vi "Main.vi"() -> ()   [LabVIEW 2020]
doc: "This template is for the Queued Message Handler design pattern.\n\nThe Event Handling Loop generates messages based on user interface actions.\n\nThe Message Handling Loop processes messages generated by the Event Handling Loop, or by other messages. The messages are string values, so new messages can be added easily to the Message Cases case structure in the Message Handling Loop. Each message cluster can also provide an optional value for Message Data, which is a variant that can be converted to whatever message-specific data is required."
uses:
  controls/WashIndicators.ctl
  controls/WashOptions.ctl
  controls/UI Data.ctl
  support/Message Queue/Message Queue.lvlib
  support/User Event - Stop/User Event - Stop.lvlib
panel:
  in  "Wash Options":T1
  out "Car Wash Indicators 2":T2
  in  "Car Position Slider":u16(slide) scale=0.0..4.0
  out "Wash Entry":bool
  out "Elapsed Time":dbl format="%<%H:%M:%S>t"
  in  "Start":bool
  in  "Stop":bool
  # "Pre-Soak\nH-P Wash\nL-P Wax\nSpot Free Rinse"
  # "Underbody Wash\nBug Remover"
  # "Tire Shine\nAir Dry"
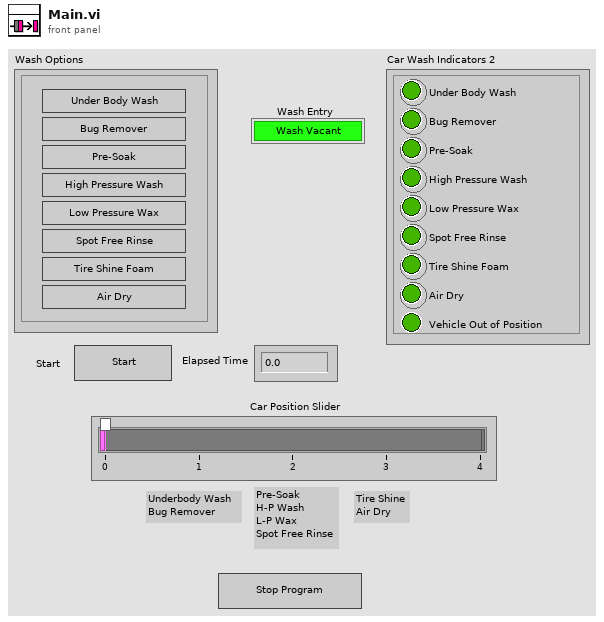
[diagram p1: front panel]
types:
  T1 = typedef "WashOptions.ctl" = cluster{"Bug Remover":bool, "Low Pressure Wax":bool, "High Pressure Wash":bool, "Pre-Soak":bool, "Spot Free Rinse":bool, "Air Dry":bool, "Under Body Wash":bool, "Tire Shine Foam":bool}
  T2 = typedef "WashIndicators.ctl" = cluster{"Bug Remover":bool, "Pre-Soak":bool, "High Pressure Wash":bool, "Spot Free Rinse":bool, "Tire Shine Foam":bool, "Low Pressure Wax":bool, "Vehicle Out of Position":bool, "Air Dry":bool, "Under Body Wash":bool}
  T3 = typedef "UI Data.ctl" = cluster{"Elapsed Time":refnum<vi>, "Wash Entry":refnum<vi>, "Car Position Slider":refnum<vi>, "Wash Options":refnum<vi>, "Car Wash Indicators":refnum<vi>, "Car Wash Indicators 2":T2}
  T4 = typedef "Message Queue.lvlib/All Message Queues.ctl" = cluster{"UI":refnum<queue>, "Status Loop":refnum<queue>}
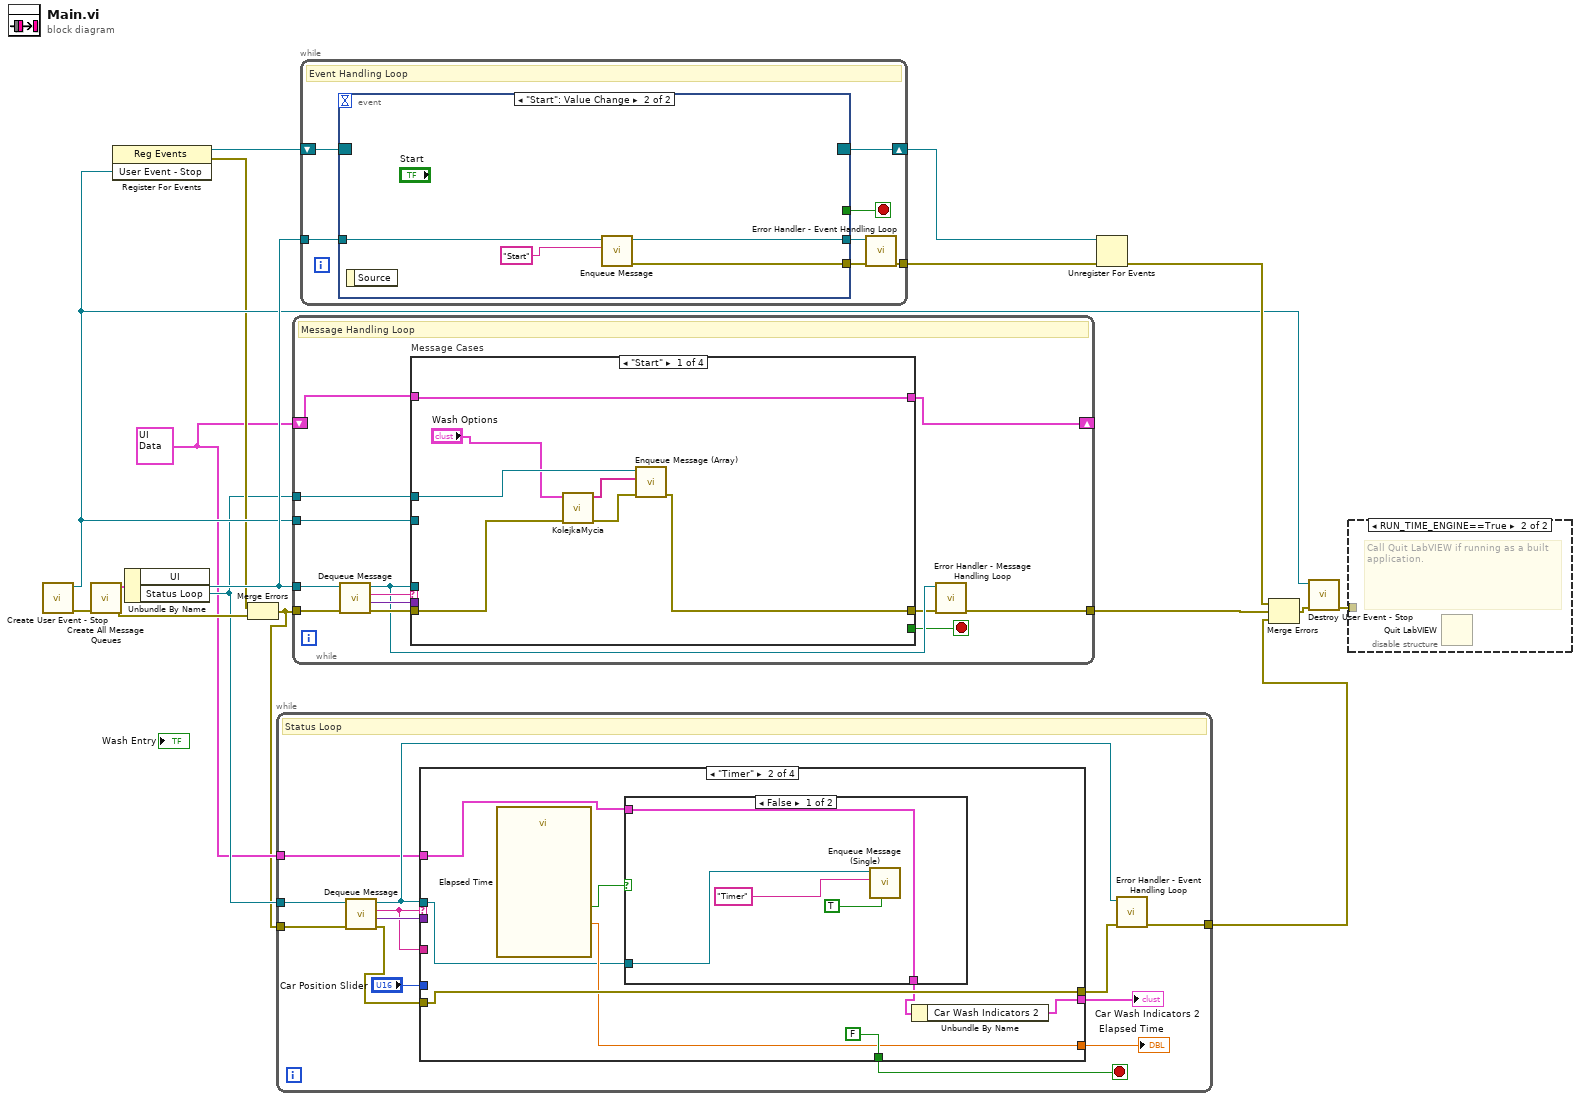
[diagram p0: block diagram]
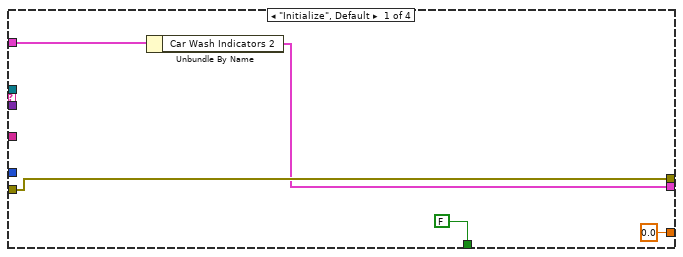
[diagram p2: hidden frame]
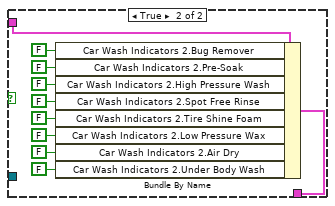
[diagram p3: hidden frame]
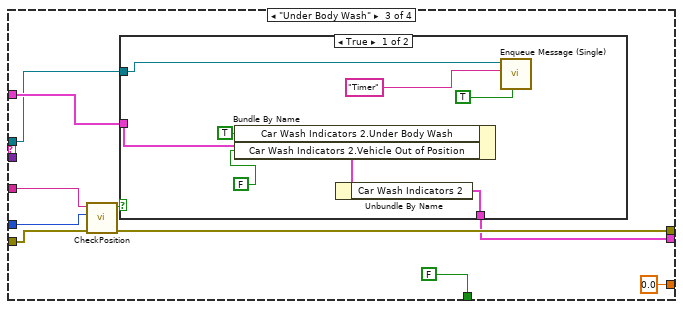
[diagram p4: hidden frame]
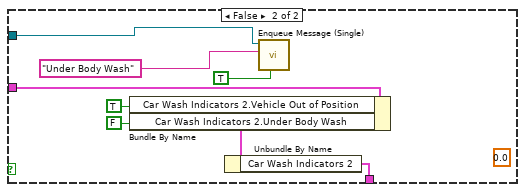
[diagram p5: hidden frame]
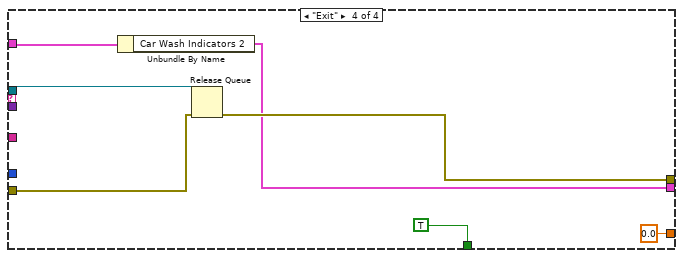
[diagram p6: hidden frame]
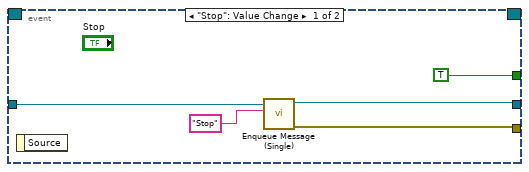
[diagram p8: hidden frame]
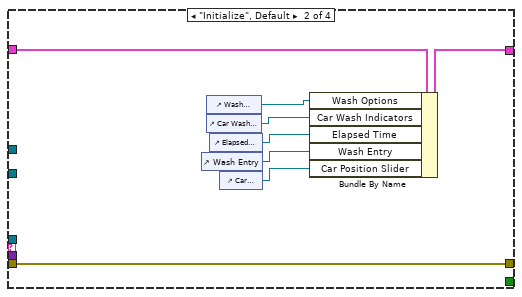
[diagram p9: hidden frame]
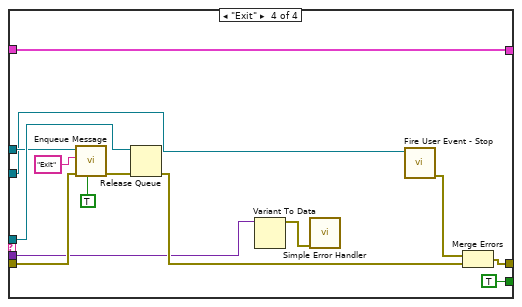
[diagram p11: hidden frame]
diagram:
  w2 = T3 {"Elapsed Time"=refnum, "Wash Entry"=refnum, "Car Position Slider"=refnum, "Wash Options"=refnum, "Car Wash Indicators"=refnum, "Car Wash Indicators 2"={"Bug Remover"=FALSE, "Pre-Soak"=FALSE, "High Pressure Wash"=FALSE, "Spot Free Rinse"=FALSE, "Tire Shine Foam"=FALSE, "Low Pressure Wax"=FALSE, "Vehicle Out of Position"=FALSE, "Air Dry"=FALSE, "Under Body Wash"=FALSE}} ("Data Cluster")
  n1 = call "Create User Event - Stop.vi"() -> ("error out"=w13:errorcluster, "User Event - Stop"=w6:refnum<user-event>)  [unwired: 10 in]
  n2 = call "Create All Message Queues.vi"("error in (no error)"=w13) -> ("error out"=w17:errorcluster, "Message Queues out"=w16:T4)  [unwired: 9 in]
  n3 = register-events(w6) -> (reference out=w7:refnum<event-registration>, error out=w5:errorcluster)  [unwired: 2 in]
  n4 = Unbundle By Name(w16) -> ("UI"=w14:refnum<queue>, "Status Loop"=w3:refnum<queue>)
  n5 = Merge Errors(w5, w17) -> (w1:errorcluster)
  n6 = while {
    tunnel: w3 -> [w30]
    tunnel: w1 -> [w29]
    tunnel: [w26] -> w4
    tunnel: w2 -> [w24]
    stop <- w23 stop-if-true
    # "Status Loop"
    n7 = call "Dequeue Message.vi"("error in (no error)"=w29, "Message Queue"=w30) -> ("error out"=w20:errorcluster, "Message Data"=w28:variant, "Message"=w21:string, "dup Message Queue"=w25:refnum<queue>)  [unwired: 6 in]
    n8 = case shown="\"Timer\"" w21 {
      tunnel: w25 -> [_ w36 w59 w90]
      tunnel: w28 -> [_ _ _ _]
      tunnel: [w34 w42 w63 w89] -> w27
      tunnel: w24 -> [w33 w38 w62 w86]
      tunnel: [FALSE FALSE FALSE TRUE] -> w23
      tunnel: "Car Position Slider" -> [_ _ w65 _]
      tunnel: w21 -> [_ _ w66 _]
      tunnel: w20 -> [w34 w42 w64 w87]
      tunnel: [w32 w39 w60 w85] -> w19
      tunnel: [0.0 ("Elapsed Time (s)") w37 0.0 ("Elapsed Time (s)") 0.0 ("Elapsed Time (s)")] -> w18
      frame "Initialize", Default {
        n9 = Unbundle By Name(w33) -> ("Car Wash Indicators 2"=w32:T2)
      }
      frame "Timer" {
        n10 = call "Elapsed Time"() -> ("Elapsed Time (s)"=w37:dbl, "Time has Elapsed"=w41:bool)  [unwired: 12 in, 6 out]
        n11 = case shown="False" w41 {
          tunnel: [w47 w49] -> w40
          tunnel: w38 -> [w47 w48]
          tunnel: w36 -> [w44 _]
          frame False {
            n12 = call "Enqueue Message (Single).vi"("Priority Message? (F)"=TRUE, "Message"="Timer", "Message Queue"=w44) -> ()  [unwired: 7 in, 2 out]
          }
          frame True {
            n13 = Bundle By Name(cluster=w48, "Car Wash Indicators 2.Bug Remover"=FALSE ("Bug Remover"), "Car Wash Indicators 2.Pre-Soak"=FALSE ("Pre-Soak"), "Car Wash Indicators 2.High Pressure Wash"=FALSE ("High Pressure Wash"), "Car Wash Indicators 2.Spot Free Rinse"=FALSE ("Spot Free Rinse"), "Car Wash Indicators 2.Tire Shine Foam"=FALSE ("Tire Shine Foam"), "Car Wash Indicators 2.Low Pressure Wax"=FALSE ("Low Pressure Wax"), "Car Wash Indicators 2.Air Dry"=FALSE ("Air Dry"), "Car Wash Indicators 2.Under Body Wash"=FALSE ("Under Body Wash")) -> (w49:T3)
          }
        }
        n14 = Unbundle By Name(w40) -> ("Car Wash Indicators 2"=w39:T2)
      }
      frame "Under Body Wash" {
        n15 = call "CheckPosition.vi"("error in"=w64, "Car Position"=w65, "State"=w66) -> ("error out"=w63:errorcluster, "Pozycja"=w61:bool)  [unwired: 7 in]
        n16 = case shown="True" w61 {
          tunnel: w62 -> [w75 w83]
          tunnel: [w73 w81] -> w60
          tunnel: w59 -> [w68 w78]
          frame True {
            n17 = Bundle By Name(cluster=w75, "Car Wash Indicators 2.Under Body Wash"=TRUE, "Car Wash Indicators 2.Vehicle Out of Position"=FALSE) -> (w74:T3)
            n18 = Unbundle By Name(w74) -> ("Car Wash Indicators 2"=w73:T2)
            n19 = call "Enqueue Message (Single).vi"("Priority Message? (F)"=TRUE, "Message"="Timer", "Message Queue"=w68) -> ()  [unwired: 7 in, 2 out]
          }
          frame False {
            (unwired) 0.0 ("Elapsed Time (s)")
            n20 = Bundle By Name(cluster=w83, "Car Wash Indicators 2.Vehicle Out of Position"=TRUE, "Car Wash Indicators 2.Under Body Wash"=FALSE) -> (w82:T3)
            n21 = Unbundle By Name(w82) -> ("Car Wash Indicators 2"=w81:T2)
            n22 = call "Enqueue Message (Single).vi"("Priority Message? (F)"=TRUE, "Message"="Under Body Wash", "Message Queue"=w78) -> ()  [unwired: 7 in, 2 out]
          }
        }
      }
      frame "Exit" {
        n23 = Unbundle By Name(w86) -> ("Car Wash Indicators 2"=w85:T2)
        n24 = Release Queue(queue=w90, error in (no error)=w87) -> (error out=w89:errorcluster)  [unwired: 1 in, 2 out]
      }
    }
    "Car Wash Indicators 2" <- w19
    "Elapsed Time" <- w18
    n25 = call "Error Handler - Event Handling Loop.vi"("error in (no error)"=w27, "Message Queue"=w25) -> ("dup error in"=w26:errorcluster)  [unwired: 8 in, 1 out]
  }
  n26 = while {
    tunnel: w14 -> [w97]
    shift-right: [w91] -> _
    shift-left: w2 -> [w103]
    tunnel: w6 -> [w102]
    tunnel: w1 -> [w101]
    tunnel: [w95] -> w15
    tunnel: w3 -> [w92]
    stop <- w93 stop-if-true
    # "Message Handling Loop"
    n27 = call "Dequeue Message.vi"("error in (no error)"=w101, "Message Queue"=w97) -> ("error out"=w100:errorcluster, "Message Data"=w98:variant, "Message"=w99:string, "dup Message Queue"=w96:refnum<queue>)  [unwired: 6 in]
    n28 = case "Message Cases" shown="\"Start\"" w99 {
      tunnel: w96 -> [_ _ _ w131]
      tunnel: w100 -> [w110 w116 w119 w133]
      tunnel: [w105 w116 w119 w134] -> w94
      tunnel: w103 -> [w106 w118 w120 w121]
      tunnel: [w106 w117 w120 w121] -> w91
      tunnel: [_ _ _ TRUE] -> w93
      tunnel: w98 -> [_ _ _ w125]
      tunnel: w102 -> [_ _ _ w126]
      tunnel: w92 -> [w109 _ _ w130]
      frame "Start" {
        # "Initialize - All initialization work should take place in this message, since other loops can potentially enqueue messages that execute immediately after this one."
        n29 = call "KolejkaMycia.vi"("error in (no error)"=w110, "Wash Options"="Wash Options") -> ("error out"=w107:errorcluster, "Option Array"=w108:string[])  [unwired: 8 in]
        n30 = call "Enqueue Message (Array).vi"("error in (no error)"=w107, "Message Array"=w108, "Message Queue"=w109) -> ("error out"=w105:errorcluster)  [unwired: 7 in, 1 out]
      }
      frame "Initialize", Default {
        # "Initialize - All initialization work should take place in this message, since other loops can potentially enqueue messages that execute immediately after this one."
        n31 = control-ref of="Wash Entry"() -> (w114:refnum<vi>)
        n32 = control-ref of="Wash Options"() -> (w111:refnum<vi>)
        n33 = control-ref of="Car Wash Indicators 2"() -> (w112:refnum<vi>)
        n34 = control-ref of="Elapsed Time"() -> (w115:refnum<vi>)
        n35 = control-ref of="Car Position Slider"() -> (w113:refnum<vi>)
        n36 = Bundle By Name(cluster=w118, "Wash Options"=w111, "Car Wash Indicators"=w112, "Elapsed Time"=w115, "Wash Entry"=w114, "Car Position Slider"=w113) -> (w117:T3)
      }
      frame "Stop" {
        # "Something - Replace this message with functionality for your own application."
      }
      frame "Exit" {
        # "Something - Replace this message with functionality for your own application."
        n37 = call-poly "Enqueue Message.vi"("Priority Message? (F)"=TRUE, "error in (no error)"=w133, "Message"="Exit", "Message Queue"=w130) -> ("error out"=w132:errorcluster)  [unwired: 6 in, 1 out]
        n38 = Release Queue(queue=w131, error in (no error)=w132) -> (error out=w128:errorcluster)  [unwired: 1 in, 2 out]
        n39 = Variant To Data(Variant=w125) -> (data=w124:errorcluster)  [unwired: 2 in, 1 out]
        n40 = call <vilib>:"Simple Error Handler.vi"("error in (no error)"=w124) -> ()  [unwired: 4 in, 5 out]
        n41 = call "Fire User Event - Stop.vi"("User Event - Stop"=w126) -> ("error out"=w127:errorcluster)  [unwired: 10 in]
        n42 = Merge Errors(w127, w128) -> (w134:errorcluster)
      }
    }
    n43 = call "Error Handler - Message Handling Loop.vi"("error in (no error)"=w94, "Message Queue"=w96) -> ("dup error in"=w95:errorcluster)  [unwired: 8 in, 1 out]
  }
  n44 = while {
    tunnel: w14 -> [w141]
    shift-right: [w139] -> w10
    shift-left: w7 -> [w140]
    tunnel: [w137] -> w8
    stop <- w135 stop-if-true
    # "Event Handling Loop"
    n45 = event shown="[1] \"Start\": Value Change" {
      selector: w140 -> [_ _]
      dyn-events: [_ _] -> w139
      timeout: _ -> [_ _]
      tunnel: w141 -> [w146 w149]
      tunnel: [w145 w147] -> w138
      tunnel: [w143 w148] -> w136
      tunnel: [TRUE _] -> w135
      event "Stop": Value Change {
        n46 = event-data() -> ()  [unwired: 1 in, 1 out]
        n47 = call "Enqueue Message (Single).vi"("Message"="Stop", "Message Queue"=w146) -> ("error out"=w143:errorcluster, "dup Message Queue"=w145:refnum<queue>)  [unwired: 8 in]
      }
      event "Start": Value Change {
        n48 = event-data() -> ()  [unwired: 1 in, 1 out]
        n49 = call-poly "Enqueue Message.vi"("Message"="Start", "Message Queue"=w149) -> ("error out"=w148:errorcluster, "dup Message Queue"=w147:refnum<queue>)  [unwired: 8 in]
      }
    }
    n50 = call "Error Handler - Event Handling Loop.vi"("error in (no error)"=w136, "Message Queue"=w138) -> ("dup error in"=w137:errorcluster)  [unwired: 8 in, 1 out]
  }
  n51 = Unregister For Events(event registration refnum=w10, error in=w8) -> (error out=w11:errorcluster)
  n52 = Merge Errors(w11, w15, w4) -> (w12:errorcluster)
  n53 = call "Destroy User Event - Stop.vi"("error in (no error)"=w12, "User Event - Stop"=w6) -> ("error out"=w9:errorcluster)  [unwired: 9 in]
  n54 = disable-structure shown="RUN_TIME_ENGINE==True" {
    disable-tunnel: w9 -> [_ _]
    frame condition #0 (active) {
    }
    frame condition #1 {
      # "Call Quit LabVIEW if running as a built application."
      n55 = Quit LabVIEW() -> ()  [unwired: 1 in]
    }
  }
